vi "Actor1_BasicNoLib_G4_4.0.0_Create.vi"(8 "error in (no error)":errorcluster, 11 "reference in":refnum<class "Actor1_BasicNoLib_G4_4.0.0.lvclass">) -> (0 "error out":errorcluster, 3 "reference out":refnum<class "Actor1_BasicNoLib_G4_4.0.0.lvclass">)   [LabVIEW 2014, in "Actor1_BasicNoLib_G4_4.0.0.lvclass"]
uses:
  <resource>/Framework/Providers/Open_GDS/ClassProviders/ActorFramework/4.0.0/Actor1_BasicNoLib_G4_4.0.0/Actor1_BasicNoLib_G4_4.0.0_class/Actor1_BasicNoLib_G4_4.0.0.lvclass
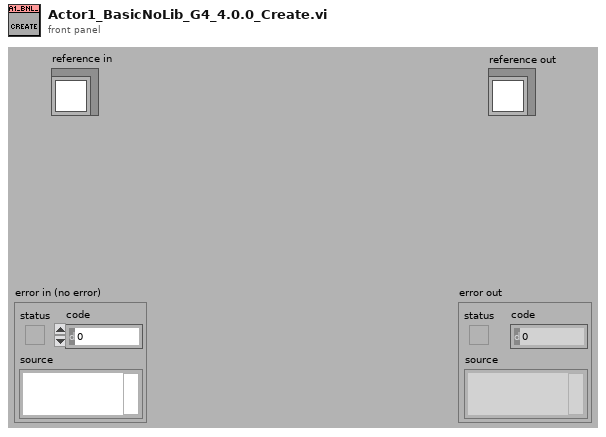
[diagram p1: front panel]
types:
  T1 = typedef "Actor1_Basic_G4_3.0.7.lvlib/Actor1_GUI_G4_3.0.7.lvclass/ObjectAttributes.ctl" = cluster{"None":bool}
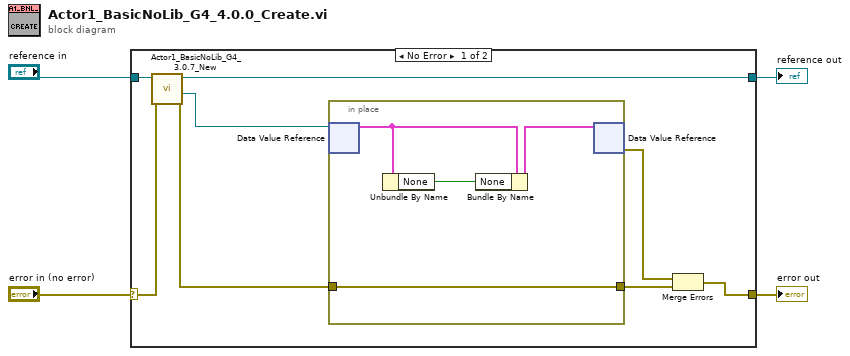
[diagram p0: block diagram]
diagram:
  n1 = case shown="No Error" "error in (no error)" {
    selector: "error in (no error)" -> [w11 w18]
    tunnel: [w8 w18] -> w3
    tunnel: "reference in" -> [w12 w17]
    tunnel: [w10 w17] -> w1
    frame No Error {
      n2 = call <resource>:"Actor1_BasicNoLib_G4_3.0.7_New.vi"("error in (no error)"=w11, "reference in"=w12) -> ("error out"=w6:errorcluster, "DVRRefOut"=w7:refnum<data-value>, "reference out"=w10:refnum<class "Actor1_BasicNoLib_G4_4.0.0.lvclass">)  [unwired: 6 in, 1 out]
      n3 = in-place {
        in-place-border: w6 -> [w13]
        in-place-border: [w13] -> w5
        n4 = in-place-dvr #1(w7) -> (w15:T1)  [unwired: 1 out]
        n5 = Unbundle By Name(w15) -> ("None"=w14:bool)
        n6 = Bundle By Name(cluster=w15, "None"=w14) -> (w16:T1)
        n7 = in-place-dvr #1(w16) -> (w9:errorcluster)  [unwired: 1 out]
      }
      n8 = Merge Errors(w9, w5) -> (w8:errorcluster)
    }
    frame Error {
    }
  }
  "error out" <- w3
  "reference out" <- w1
